vi "get values.vi"(11 "USB In":string) -> (1 "insidex (0-319)":dbl, 2 "averagex (0-319)":dbl, 3 "status":dbl)   [LabVIEW 2019]
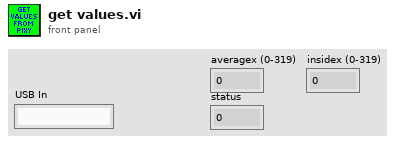
[diagram p1: front panel]
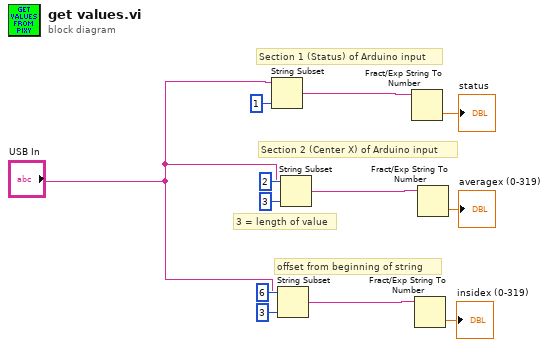
[diagram p0: block diagram]
diagram:
  # "offset from beginning of string"
  # "3 = length of value"
  # "Section 2 (Center X) of Arduino input"
  # "Section 1 (Status) of Arduino input"
  n1 = String Subset(string="USB In", length (rest)=1 ("length (rest)")) -> (substring=w11:string)  [unwired: 1 in]
  n2 = String Subset(string="USB In", offset (0)=6, length (rest)=3 ("length (rest)")) -> (substring=w5:string)
  n3 = String Subset(string="USB In", offset (0)=2, length (rest)=3 ("length (rest)")) -> (substring=w10:string)
  n4 = Fract/Exp String To Number(string=w11) -> (number=→"status":dbl)  [unwired: 3 in, 1 out]
  n5 = Fract/Exp String To Number(string=w5) -> (number=→"insidex (0-319)":dbl)  [unwired: 3 in, 1 out]
  n6 = Fract/Exp String To Number(string=w10) -> (number=→"averagex (0-319)":dbl)  [unwired: 3 in, 1 out]
